vi "LWXPS_EEPROMDACOffsetCIESet.vi"(0 "XPS Reference IN":refnum<k24>, 5 "Plug Number":i32, 7 "DAC1 Offset":dbl, 9 "DAC2 Offset":dbl, 11 "LabVIEW error IN":errorcluster) -> (4 "XPS Reference OUT":refnum<k24>, 6 "Returned error code":i32, 8 "XPS Error String":string, 15 "LabVIEW error OUT":errorcluster)   [LabVIEW 2014]
uses:
  D:/XPSQ8_LabView_Library/Development/Source/Dll/Newport.XPS.CommandInterface.dll
  Dll/Newport.XPS.CommandInterface.dll
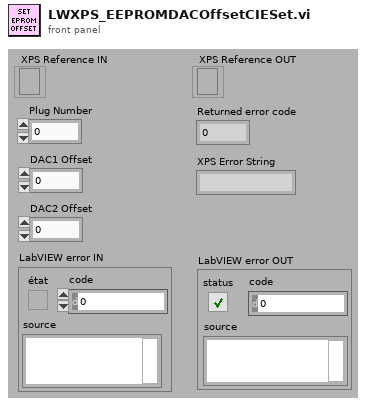
[diagram p1: front panel]
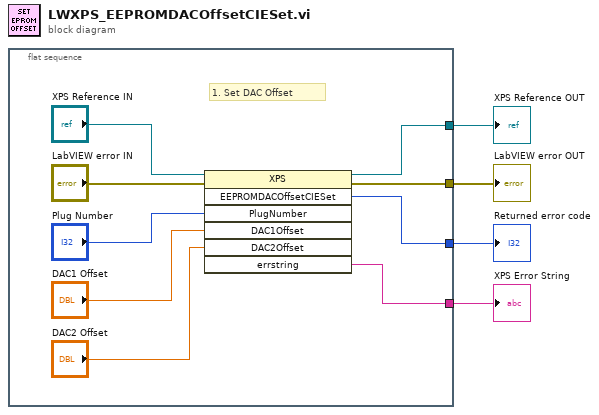
[diagram p0: block diagram]
diagram:
  n1 = flat-sequence {
    tunnel: [w10] -> w4
    tunnel: [w13] -> w3
    tunnel: [w9] -> w2
    tunnel: [w7] -> w1
    frame #0 {
      # "1. Set DAC Offset"
      n2 = invoke class="XPS" method="EEPROMDACOffsetCIESet"(reference="XPS Reference IN", error in="LabVIEW error IN", "PlugNumber"="Plug Number", "DAC1Offset"="DAC1 Offset", "DAC2Offset"="DAC2 Offset") -> (reference out=w10:refnum<k24>, error out=w13:errorcluster, "EEPROMDACOffsetCIESet"=w9:i32, "errstring"=w7:string)  [unwired: 2 in, 3 out]
    }
  }
  "XPS Reference OUT" <- w4
  "LabVIEW error OUT" <- w3
  "Returned error code" <- w2
  "XPS Error String" <- w1
